vi "Sort_Tone_Errors.vi"(10 "Array 3":T1[](array[typedef]), 11 "Array in":i32[](array[numeric])) -> (3 "Array out":T1[](array[typedef]))   [LabVIEW 2018]
uses:
  Controls/Clusts/ErrorStatus.ctl
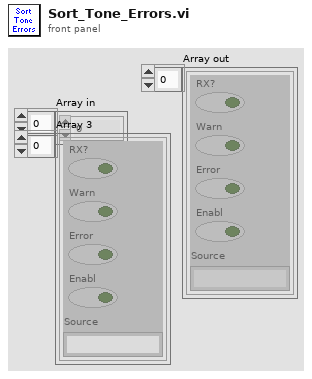
[diagram p1: front panel]
types:
  T1 = typedef "ErrorStatus.ctl" = cluster{"RX?":bool, "Warn":bool, "Error":bool, "Enabl":bool, "Source":string}
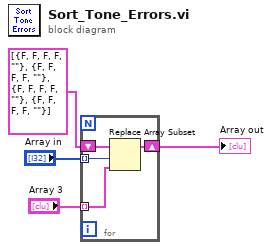
[diagram p0: block diagram]
diagram:
  n1 = for {
    tunnel: "Array 3" -> [w7] mode=indexing
    tunnel: "Array in" -> [w6] mode=indexing
    shift-right: [w5] -> w4
    shift-left: T1[] [{"RX?"=FALSE, "Warn"=FALSE, "Error"=FALSE, "Enabl"=FALSE, "Source"=""}, {"RX?"=FALSE, "Warn"=FALSE, "Error"=FALSE, "Enabl"=FALSE, "Source"=""}, {"RX?"=FALSE, "Warn"=FALSE, "Error"=FALSE, "Enabl"=FALSE, "Source"=""}, {"RX?"=FALSE, "Warn"=FALSE, "Error"=FALSE, "Enabl"=FALSE, "Source"=""}] -> [w8]
    n2 = Replace Array Subset(array=w8, new element=w7, index=w6) -> (w5:T1[])
  }
  "Array out" <- w4
